vi "Modif-meteo-param.vi"(1 "input cluster":T1) -> (0 "output cluster":T1)   [LabVIEW 2010]
panel:
  in  "cancel":bool
  in  "ok":bool
  in  "Température Minimale":dbl=-35.0 format="%.2g"
  in  "Vélocité maximale":dbl=50.0 format="%.2g"
  in  "échelle de temps (minutes)":dbl=0.5 format="%.2g"
  in  "Variation en %":dbl=2.0 format="%.2g"
  in  "échelle de temps (minutes)":dbl=30.0 format="%.2g"
  in  "humidité maximale":dbl=90.0 format="%.2g"
  in  "Variation en °C":dbl=2.0 format="%.2g"
  in  "Température Maximale":dbl=35.0 format="%.2g"
  in  "sécurité en °C":dbl=1.0 format="%.2g"
  in  "Alarme point de rosée":bool=TRUE
  in  "Alarme D température":bool=TRUE
  in  "Alarme vent":bool=TRUE
  in  "Alarme D humidité":bool=TRUE
  in  "Alarme Température":bool=TRUE
  in  "Alarme Humidité":bool=TRUE
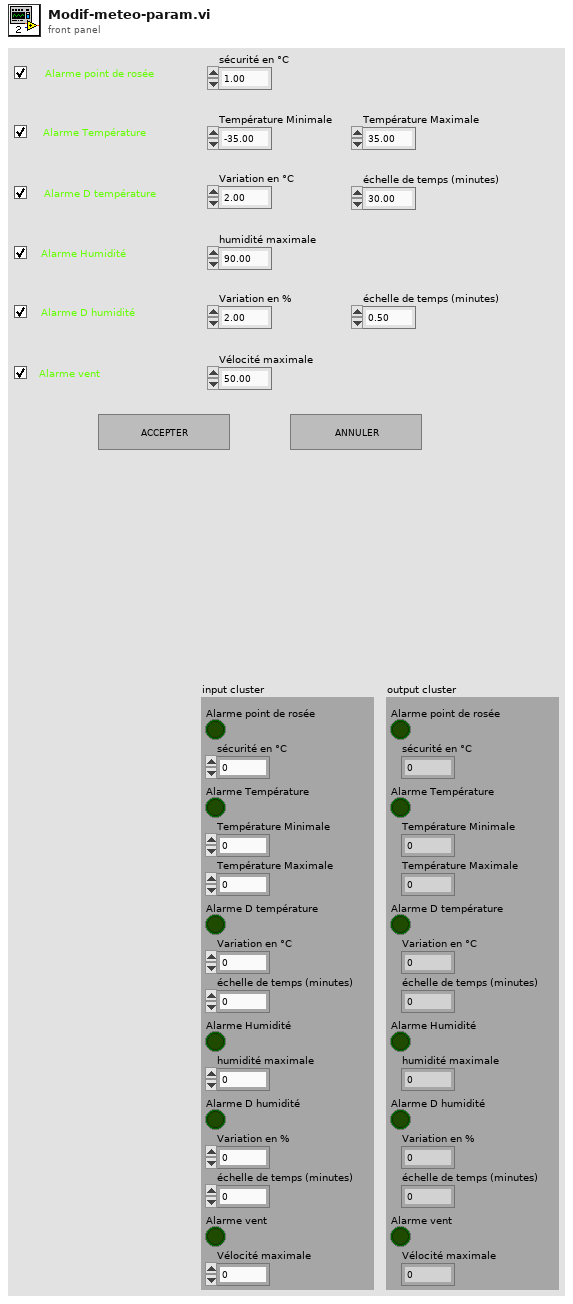
[diagram p1: front panel]
types:
  T1 = cluster{"Alarme point de rosée":bool, "sécurité en °C":dbl, "Alarme Température":bool, "Température Minimale":dbl, "Température Maximale":dbl, "Alarme D température":bool, "Variation en °C":dbl, "échelle de temps (minutes)":dbl, "Alarme Humidité":bool, "humidité maximale":dbl, "Alarme D humidité":bool, "Variation en %":dbl, "échelle de temps (minutes)":dbl, "Alarme vent":bool, "Vélocité maximale":dbl}
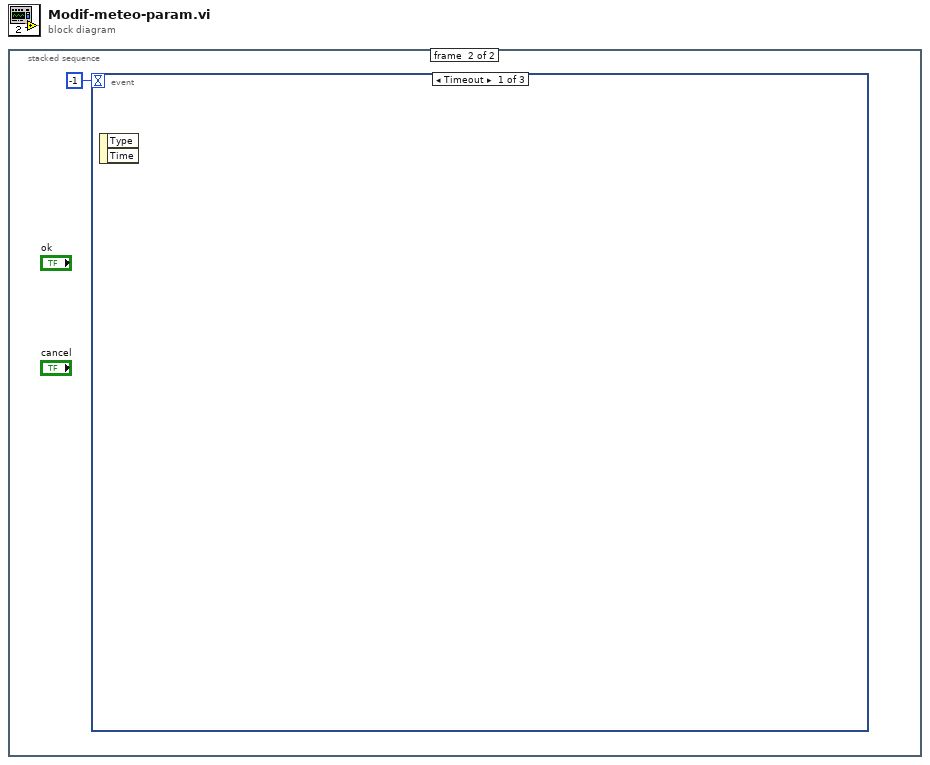
[diagram p0: block diagram]
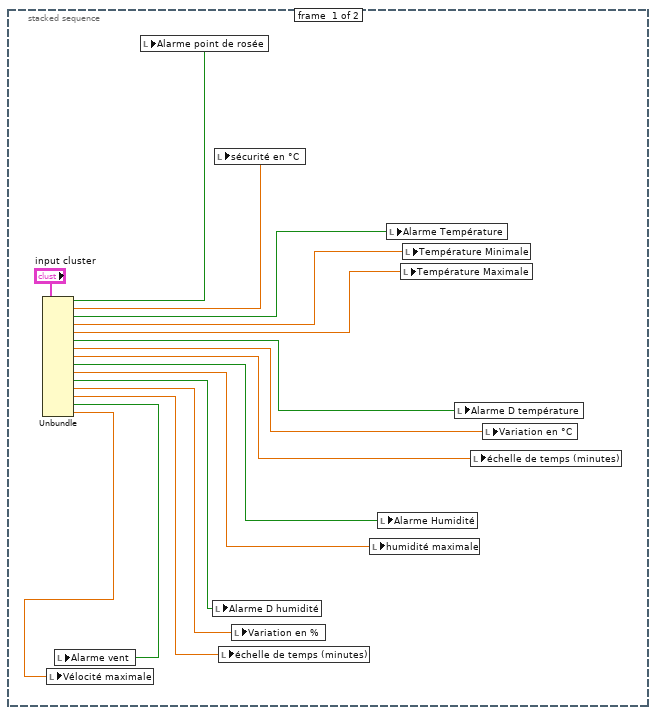
[diagram p2: hidden frame]
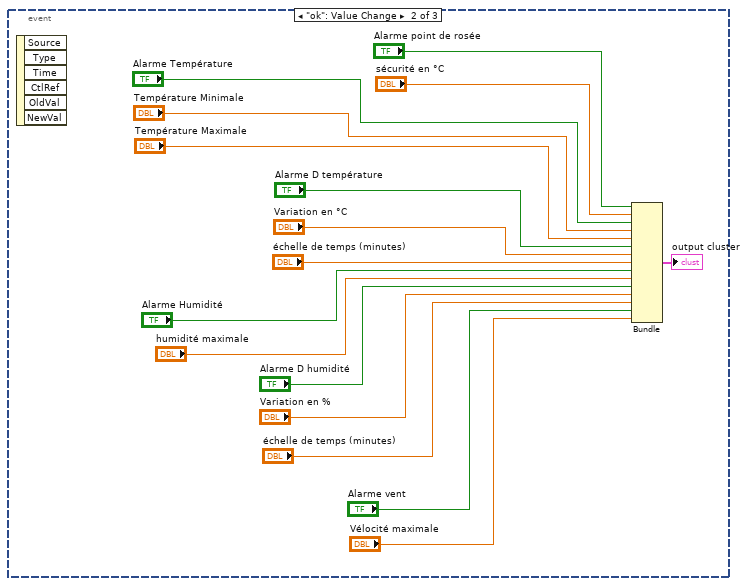
[diagram p3: hidden frame]
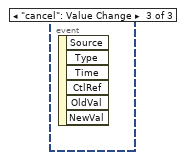
[diagram p4: hidden frame]
diagram:
  n1 = stacked-sequence {
    frame #0 {
      n2 = Unbundle("input cluster") -> ("Alarme point de rosée"=w1:bool, "sécurité en °C"=w2:dbl, "Alarme Température"=w3:bool, "Température Minimale"=w4:dbl, "Température Maximale"=w5:dbl, "Alarme D température"=w6:bool, "Variation en °C"=w7:dbl, "échelle de temps (minutes)"=w8:dbl, "Alarme Humidité"=w10:bool, "humidité maximale"=w9:dbl, "Alarme D humidité"=w13:bool, "Variation en %"=w12:dbl, "échelle de temps (minutes)"=w11:dbl, "Alarme vent"=w15:bool, "Vélocité maximale"=w14:dbl)
      n3 = local write "Vélocité maximale"(w14) -> ()
      n4 = local write "Alarme vent"(w15) -> ()
      n5 = local write "Alarme point de rosée"(w1) -> ()
      n6 = local write "Alarme D humidité"(w13) -> ()
      n7 = local write "sécurité en °C"(w2) -> ()
      n8 = local write "échelle de temps (minutes)"(w11) -> ()
      n9 = local write "Variation en %"(w12) -> ()
      n10 = local write "humidité maximale"(w9) -> ()
      n11 = local write "Alarme Humidité"(w10) -> ()
      n12 = local write "Alarme Température"(w3) -> ()
      n13 = local write "Température Maximale"(w5) -> ()
      n14 = local write "Température Minimale"(w4) -> ()
      n15 = local write "Alarme D température"(w6) -> ()
      n16 = local write "échelle de temps (minutes)"(w8) -> ()
      n17 = local write "Variation en °C"(w7) -> ()
    }
    frame #1 {
      n18 = event shown="[0] Timeout" {
        selector: _ -> [_ _ _]
        dyn-events: _ -> [_ _ _]
        timeout: -1 -> [_ _ _]
        event Timeout {
          n19 = event-data() -> ()  [unwired: 1 in, 2 out]
        }
        event "ok": Value Change {
          n20 = event-data() -> ()  [unwired: 1 in, 6 out]
          n21 = Bundle("Alarme point de rosée"="Alarme point de rosée", "sécurité en °C"="sécurité en °C", "Alarme Température"="Alarme Température", "Température Minimale"="Température Minimale", "Température Maximale"="Température Maximale", "Alarme D température"="Alarme D température", "Variation en °C"="Variation en °C", "échelle de temps (minutes)"="échelle de temps (minutes)", "Alarme Humidité"="Alarme Humidité", "humidité maximale"="humidité maximale", "Alarme D humidité"="Alarme D humidité", "Variation en %"="Variation en %", "échelle de temps (minutes)"="échelle de temps (minutes)", "Alarme vent"="Alarme vent", "Vélocité maximale"="Vélocité maximale") -> (→"output cluster":T1)  [unwired: 1 in]
        }
        event "cancel": Value Change {
          n22 = event-data() -> ()  [unwired: 1 in, 6 out]
        }
      }
    }
  }
